vi "PVCAMTriggerToON_OFF.vi"(11 "TriggerOut":T1) -> (3 "y":T2)   [LabVIEW 2013, in "Photometrics_CH-250_Cam.lvclass"]
uses:
  Photometrics_CH-250_Cam.lvclass
  shared/OnOffTypeDef.ctl
  TriggerMode_TypDef.ctl
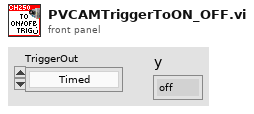
[diagram p1: front panel]
types:
  T1 = typedef "TriggerMode_TypDef.ctl" = enum16{"Timed", "Strobed", "Bulb", "Trigger first", "Flash", "Variable Timed"}
  T2 = typedef "OnOffTypeDef.ctl" = enum16{"off", "on"}
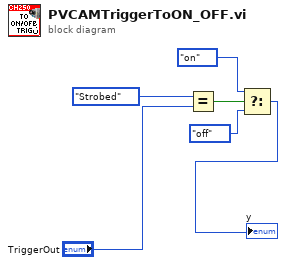
[diagram p0: block diagram]
diagram:
  n1 = Equal?(x=TriggerMode_TypDef."Strobed" ("trigger mode (input)"), y="TriggerOut") -> (x = y?=w3:bool)
  n2 = Select(t=OnOffTypeDef."on" ("y"), s=w3, f=OnOffTypeDef."off" ("y")) -> (s? t:f=→"y":T2)
